vi "Write Multiple Channels with Simple Header.vi"() -> ()   [LabVIEW 2012]
doc: "本VI按照日期和时间自动生成一个字符串，并打开以该字符串为名称的文件。包含一个正弦波和一个方波的数组被转换为制表符分隔的字符串，并写入文件。然后关闭文件。"
uses:
  <vilib>/Analysis/NI_AALBase.lvlib
panel:
  in  "UUT序列号":string="A12345"
  in  "操作员姓名":string="Leonardo DaVinci"
  out "仿真数据":dbl[][](graph)
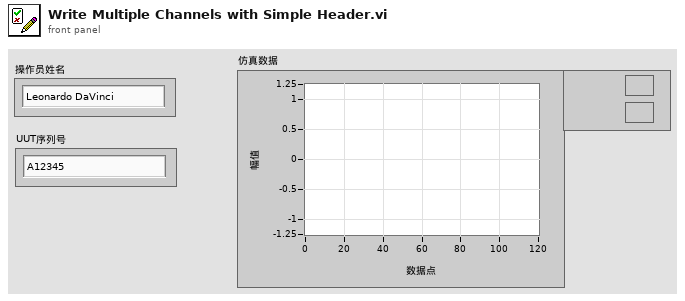
[diagram p1: front panel]
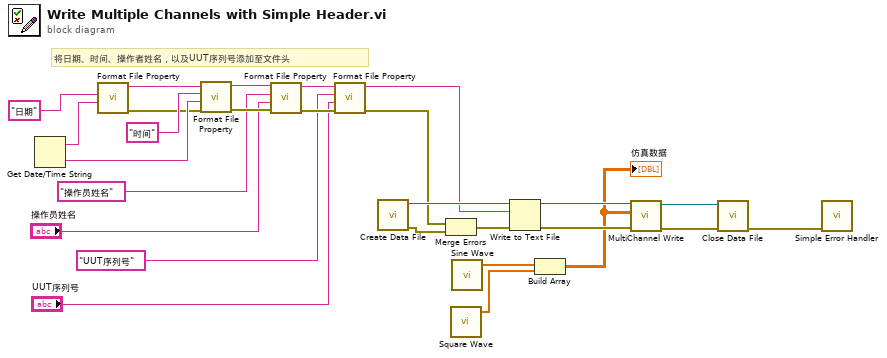
[diagram p0: block diagram]
diagram:
  # "将日期、时间、操作者姓名，以及UUT序列号添加至文件头"
  n1 = Get Date/Time String ("获取日期/时间字符串")() -> (date string=w24:string, time string=w21:string)  [unwired: 3 in]
  n2 = call "Format File Property.vi"("文件属性值"=w24, "文件属性名称"="日期") -> ("错误输出"=w14:cluster{"状态":bool, "代码":i32, "源":string}, "字符串输出"=w22:string)  [unwired: 8 in]
  n3 = call "Format File Property.vi"("错误输入"=w14, "文件属性值"=w21, "文件属性名称"="时间", "字符串输入"=w22) -> ("错误输出"=w15:cluster{"状态":bool, "代码":i32, "源":string}, "字符串输出"=w16:string)  [unwired: 6 in]
  n4 = call "Format File Property.vi"("错误输入"=w15, "文件属性值"="操作员姓名", "文件属性名称"="操作员姓名", "字符串输入"=w16) -> ("错误输出"=w13:cluster{"状态":bool, "代码":i32, "源":string}, "字符串输出"=w12:string)  [unwired: 6 in]
  n5 = call "Format File Property.vi"("错误输入"=w13, "文件属性值"="UUT序列号", "文件属性名称"="UUT序列号", "字符串输入"=w12) -> ("错误输出"=w8:cluster{"状态":bool, "代码":i32, "源":string}, "字符串输出"=w11:string)  [unwired: 6 in]
  n6 = call "Create Data File.vi"() -> ("错误输出"=w6:cluster{"状态":bool, "代码":i32, "源":string}, "文件引用句柄"=w20:refnum<file>)  [unwired: 10 in]
  n7 = Merge Errors ("合并错误")(w8, w6) -> (w7:errorcluster)
  n8 = call <vilib>:"Square Wave.vi"() -> ("square wave"=w26:dbl[])  [unwired: 6 in, 2 out]
  n9 = call <vilib>:"Sine Wave.vi"() -> ("sine wave"=w27:dbl[])  [unwired: 5 in, 2 out]
  n10 = Write to Text File ("写入文本文件")(file (use dialog)=w20, text=w11, error in=w7) -> (refnum out=w19:refnum<file>, error out=w18:errorcluster)  [unwired: 1 in, 1 out]
  n11 = Build Array ("创建数组")(w27, w26) -> (w17:dbl[][])
  "仿真数据" <- w17
  n12 = call "MultiChannel Write.vi"("错误输入"=w18, "数据至记录"=w17, "文件引用句柄输入"=w19) -> ("错误输出"=w3:cluster{"状态":bool, "代码":i32, "源":string}, "文件引用句柄输出"=w1:refnum<file>)  [unwired: 7 in]
  n13 = call "Close Data File.vi"("错误输入"=w3, "文件引用句柄输入"=w1) -> ("错误输出"=w2:errorcluster)  [unwired: 9 in]
  n14 = call <vilib>:"Simple Error Handler.vi"("error in (no error)"=w2) -> ()  [unwired: 4 in, 5 out]
